vi "CML.vi"() -> ()   [LabVIEW 2024]
uses:
  <instrlib>/OptoMMP/OptoMMP.lvlib
panel:
  in  "Channel No.":i32
  in  "stop":bool
  in  "Client IP Address":string
  out "Waveform Chart":waveform(sgl)(graph)
  out "Measurements":sgl[](array[numeric])
  # "Opto 22 Continuous Measurement"
  # "Enter the IP address of\nthe Opto 22 device"
  # "Copyright (c) 2025 California Institute of Technology (Caltech).\nU.S. Government sponsorship acknowledged.\n\nLicensed under the Apache License, Version 2.0 (the \"License\");\nyou may not use this file except in compliance with the License.\nYou may obtain a copy of the License at\n\n    http://www.apache.org/licenses/LICENSE-2.0\n\nUnless required by applicable law or agreed to in writing, software\ndistributed under the License is distributed on an \"AS IS\" BASIS,\nWITHOUT WARRANTIES OR CONDITIONS OF ANY KIND, either express or implied.\nSee the License for the specific language governing permissions and\nlimitations under the License."
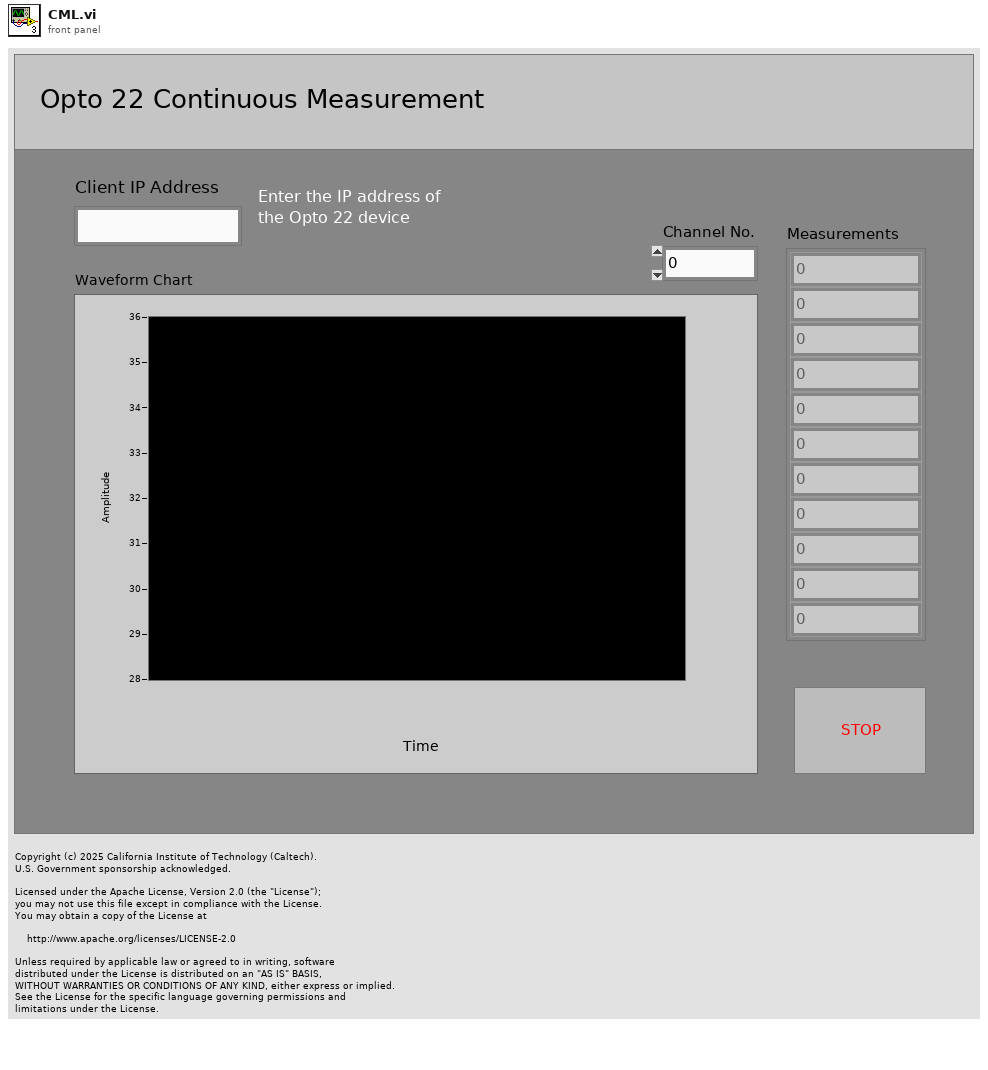
[diagram p1: front panel]
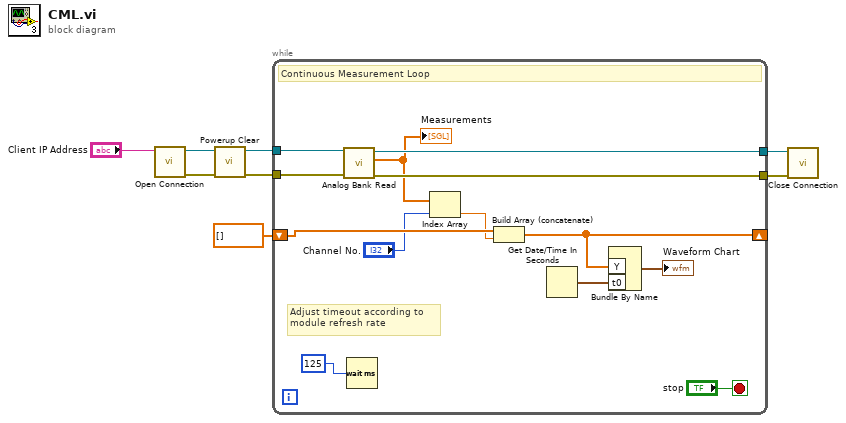
[diagram p0: block diagram]
diagram:
  n1 = call <instrlib>:"Open Connection.vi"("Client IP Address"="Client IP Address") -> ("error out"=w5:errorcluster, "TCP Network Connection out"=w6:refnum<k5>)  [unwired: 9 in]
  n2 = call <instrlib>:"Powerup Clear.vi"("error in (no error)"=w5, "TCP Network Connection in"=w6) -> ("error out"=w3:errorcluster, "connection ID out"=w4:refnum<k5>)  [unwired: 8 in]
  n3 = while {
    tunnel: w4 -> [w21]
    tunnel: w3 -> [w20]
    tunnel: [w19] -> w8
    tunnel: [w18] -> w7
    shift-right: [w12] -> _
    shift-left: sgl[] [] -> [w15]
    stop <- "stop" stop-if-true
    # "Adjust timeout according to\nmodule refresh rate"
    # "Continuous Measurement Loop"
    n4 = call <instrlib>:"Analog Bank Read.vi"("error in (no error)"=w20, "TCP Network Connection in"=w21) -> ("error out"=w18:errorcluster, "Measurements"=w10:sgl[], "TCP Network Connection out"=w19:refnum<k5>)  [unwired: 7 in]
    "Measurements" <- w10
    n5 = Wait (ms)(milliseconds to wait=u32 125) -> ()  [unwired: 1 out]
    n6 = Index Array(array=w10, index="Channel No.") -> (element=w14:sgl)
    n7 = Build Array (concatenate)(w15, w14) -> (w12:sgl[])
    n8 = Get Date/Time In Seconds() -> (seconds since 1Jan1904=w13:timestamp)
    n9 = Bundle By Name("Y"=w12, "t0"=w13) -> (→"Waveform Chart":waveform(sgl))  [unwired: 1 in]
  }
  n10 = call <instrlib>:"Close Connection.vi"("error in (no error)"=w7, "TCP Network Connection in"=w8) -> ()  [unwired: 8 in, 2 out]
